vi "testReadKeysFromConfigFile.vi"(8 "error in (no error)":errorcluster) -> (0 "error out":errorcluster)   [LabVIEW 2018]
doc: "Test the readKeysFromConfigFile.vi."
uses:
  <vilib>/addons/_JKI Toolkits/Caraya/classes/Test/Test.lvclass
  <vilib>/addons/_JKI Toolkits/Caraya/classes/Assert/Assert.lvclass
  <vilib>/addons/_JKI Toolkits/Caraya/classes/Assert/Assert Equal Type_Variant.vi
  <vilib>/Utility/config.llb/NI_LVConfig.lvlib
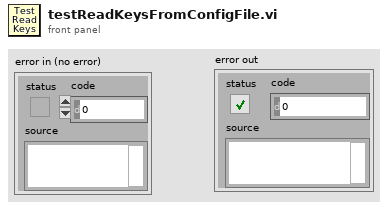
[diagram p1: front panel]
types:
  T1 = typedef "NI_LVConfig.lvlib/Config Data RefNum.ctl" = refnum<k1>
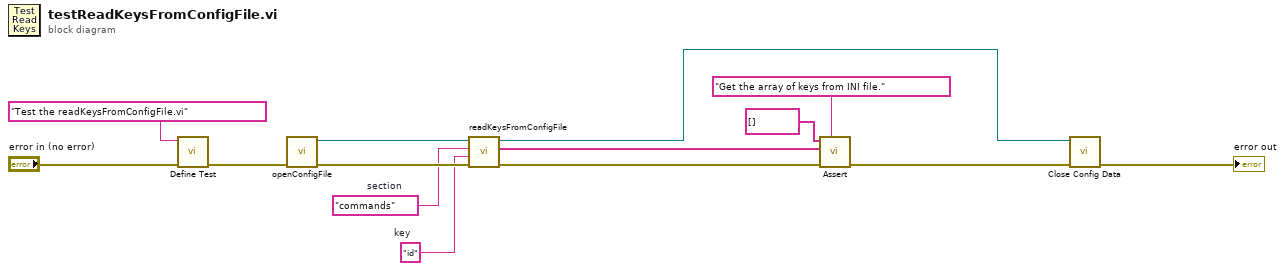
[diagram p0: block diagram]
diagram:
  w6 = "id"  # key
  w7 = "commands"  # section
  n1 = call <vilib>:"Define Test.vi"("error in (no error)"="error in (no error)", "Label (VI Title)"="Test the readKeysFromConfigFile.vi") -> ("error out"=w10:errorcluster)  [unwired: 9 in]
  n2 = call "openConfigFile.vi"("error in (no error)"=w10) -> ("error out"=w9:errorcluster, "Path out"=w8:T1)  [unwired: 9 in]
  n3 = call "readKeysFromConfigFile.vi"("error in (no error)"=w9, "key"=w6, "section"=w7, "Refnum in"=w8) -> ("error out"=w3:errorcluster, "arrayOfKeys"=w4:string[], "Refnum out"=w1:T1)  [unwired: 5 in]
  n4 = call-poly <vilib>:"Assert.vi"("Label"="Get the array of keys from INI file.", "error in (no error)"=w3, "Y"=w4, "X"=string[] []) -> ("error out"=w11:errorcluster)  [unwired: 7 in]
  n5 = call <vilib>:"Close Config Data.vi"("error in (no error)"=w11, "refnum"=w1) -> ("error out"=→"error out":errorcluster)  [unwired: 8 in, 1 out]
